vi "Shooter Ready.vi"(10 "actual":dbl, 11 "target":dbl) -> (3 "Shooter Ready?":bool)   [LabVIEW 2020]
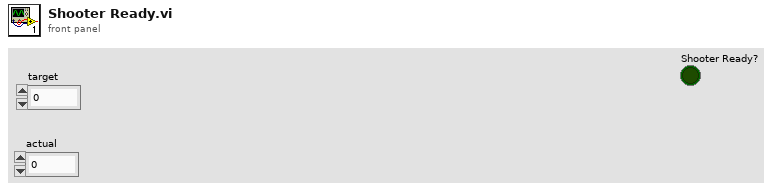
[diagram p1: front panel]
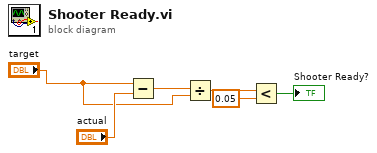
[diagram p0: block diagram]
diagram:
  n1 = Subtract(x="target", y="actual") -> (x-y=w5:dbl)
  n2 = Divide(x=w5, y="target") -> (x/y=w3:dbl)
  n3 = Less?(x=w3, y=0.05) -> (x < y?=→"Shooter Ready?":bool)
